vi "Get Param (Number).vi"(8 "error in (no error)":errorcluster, 9 "Default":dbl, 10 "Name":string, 11 "Request in":refnum<class "Request.lvclass">) -> (0 "error out":errorcluster, 1 "Value":dbl, 2 "Found?":bool, 3 "Request out":refnum<class "Request.lvclass">)   [LabVIEW 2017, in "Request.lvclass"]
uses:
  Request.lvclass
  Request.lvclass/Request.ctl
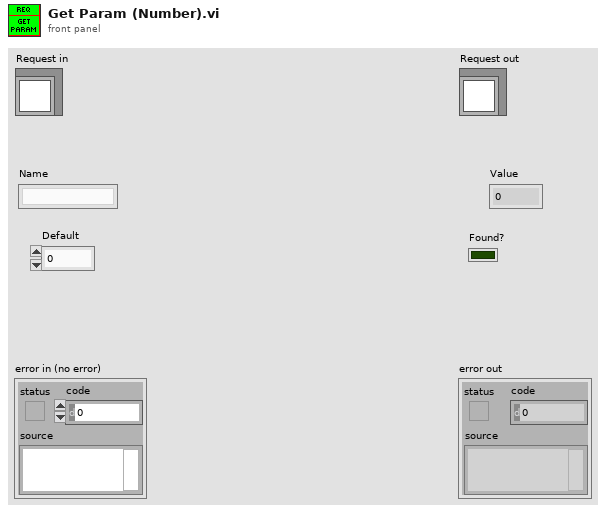
[diagram p1: front panel]
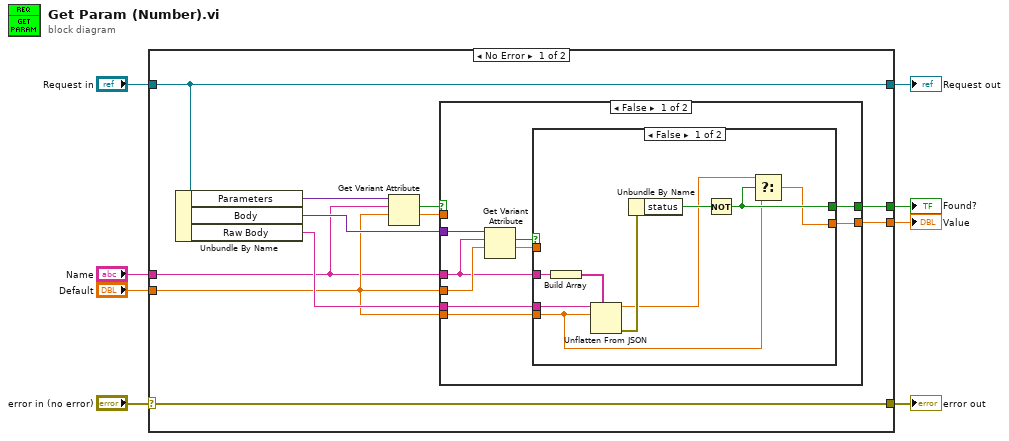
[diagram p0: block diagram]
diagram:
  n1 = case shown="No Error" "error in (no error)" {
    selector: "error in (no error)" -> [w19 w42]
    tunnel: [w19 w42] -> w7
    tunnel: [w18 w43] -> w5
    tunnel: "Request in" -> [w18 w43]
    tunnel: [w13 _] -> w4
    tunnel: "Name" -> [w9 _]
    tunnel: [w12 _] -> w2
    tunnel: "Default" -> [w10 _]
    frame No Error {
      n2 = Unbundle By Name(w18) -> ("Parameters"=w17:variant, "Body"=w15:variant, "Raw Body"=w11:string)
      n3 = Get Variant Attribute(Variant=w17, name=w9, default value (empty Variant)=w10) -> (found=w16:bool, value=w14:dbl)  [unwired: 1 in, 2 out]
      n4 = case shown="False" w16 {
        selector: w16 -> [_ w40]
        tunnel: w15 -> [w28 _]
        tunnel: w14 -> [_ w41]
        tunnel: [w25 w41] -> w13
        tunnel: [w23 w40] -> w12
        tunnel: w11 -> [w22 _]
        tunnel: w10 -> [w27 _]
        tunnel: w10 -> [w21 _]
        tunnel: w9 -> [w20 _]
        frame False {
          n5 = Get Variant Attribute(Variant=w28, name=w20, default value (empty Variant)=w27) -> (found=w26:bool, value=w24:dbl)  [unwired: 1 in, 2 out]
          n6 = case shown="False" w26 {
            selector: w26 -> [_ w38]
            tunnel: [w29 w39] -> w25
            tunnel: w24 -> [_ w39]
            tunnel: [w32 w38] -> w23
            tunnel: w22 -> [w37 _]
            tunnel: w21 -> [w31 _]
            tunnel: w20 -> [w36 _]
            frame False {
              n7 = Build Array(w36) -> (w35:string[])
              n8 = Unflatten From JSON(path=w35, JSON string=w37, type and defaults=w31) -> (value=w30:dbl, error out=w34:errorcluster)  [unwired: 4 in]
              n9 = Unbundle By Name(w34) -> ("status"=w33:bool)
              n10 = Not(x=w33) -> (.not. x?=w32:bool)
              n11 = Select(t=w30, s=w32, f=w31) -> (s? t:f=w29:dbl)
            }
            frame True {
            }
          }
        }
        frame True {
        }
      }
    }
    frame Error {
    }
  }
  "error out" <- w7
  "Request out" <- w5
  "Value" <- w4
  "Found?" <- w2
